vi "Get Data Log File Settings.vi"(8 "error in":errorcluster, 11 "File Ref in":T1 format="%.0x") -> (0 "error out":errorcluster, 1 "Example File Path":path, 2 "Log File Path":path, 3 "File Ref out":T1 format="%.0x", 5 "Name":string)   [LabVIEW 2015, in "Waveform Data Logger System Explorer.lvlib"]
uses:
  Waveform Data Logger System Explorer.lvlib
  <vilib>/NI Veristand/Custom Device API/Custom Device Item Ref.ctl
  Shared/Classes/Log File Specifications/Log File Specification/Log File Specification.lvclass
  Shared/Classes/Log File Specifications/Log File Specification/Log File Specification.lvclass/Log File Specification.ctl
  Shared/Globals/Property Strings.vi
  <vilib>/NI Veristand/Custom Device API/Get Item Property (Path).vi
  <vilib>/Utility/error.llb/Error Cluster From Error Code.vi
  <vilib>/NI VeriStand/Custom Device API/Custom Device API.lvlib
  Shared/Waveform Data Logger Shared.lvlib
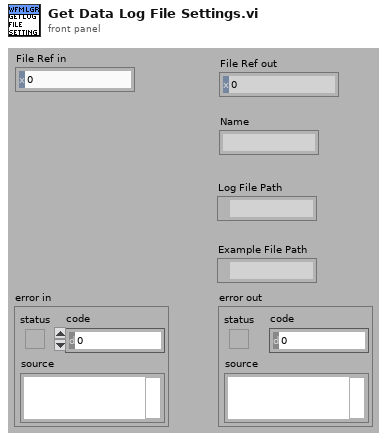
[diagram p1: front panel]
types:
  T1 = typedef "Custom Device API.lvlib/Custom Device Item Ref.ctl" = u64
  T2 = typedef "Custom Device API.lvlib/Custom Device Item Info.ctl" = cluster{"Name":string, "Is Channel":bool, "GUID":string, "Is Waveform":bool}
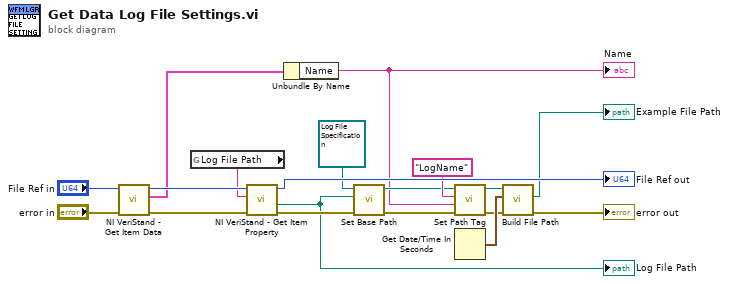
[diagram p0: block diagram]
diagram:
  n1 = call <vilib>:"NI VeriStand - Get Item Data.vi"("error in (no error)"="error in", "Item Ref in"="File Ref in") -> ("error out"=w18:errorcluster, "Item Info"=w17:T2, "Item Ref out"=w19:T1)  [unwired: 7 out]
  n2 = global read "Property Strings.vi" "Log File Path"() -> (w14:string)
  n3 = call-poly <vilib>:"NI VeriStand - Get Item Property.vi"("error in (no error)"=w18, "Property Name"=w14, "Item Ref in"=w19) -> ("error out"=w12:errorcluster, "Value"=w7:path, "Item Ref out"=→"File Ref out":T1)  [unwired: 1 in, 5 out]
  "Log File Path" <- w7
  n4 = Unbundle By Name(w17) -> ("Name"=w3:string)
  "Name" <- w3
  n5 = call "Set Base Path.vi"("error in (no error)"=w12, "Base Path"=w7, "Log File Specification in"=refnum<class "Log File Specification.lvclass"> refnum ("Waveform Data Logger Engine.lvlib:Log File Specification.lvclass")) -> ("error out"=w4:errorcluster, "Log File Specification out"=w5:refnum<class "Log File Specification.lvclass">)  [unwired: 7 in]
  n6 = call "Set Path Tag.vi"("error in (no error)"=w4, "Tag Value"=w3, "Tag Name"="LogName", "Log File Specification in"=w5) -> ("error out"=w1:errorcluster, "Log File Specification out"=w2:refnum<class "Log File Specification.lvclass">)  [unwired: 6 in]
  n7 = Get Date/Time In Seconds() -> (seconds since 1Jan1904=w10:timestamp)
  n8 = call "Build File Path.vi"("error in (no error)"=w1, "Time Stamp"=w10, "Log File Specification in"=w2) -> ("error out"=→"error out":errorcluster, "Instance File Path"=→"Example File Path":path)  [unwired: 6 in, 1 out]
